vi "Convert Relative Path.vi"(8 "error in (no error)":errorcluster, 10 "File Path in":path, 11 "Report Plugin.lvclass 2":refnum<class "Report Plugin.lvclass">) -> (0 "error out":errorcluster, 2 "Modified Path":path, 3 "Report Plugin.lvclass":refnum<class "Report Plugin.lvclass">)   [LabVIEW 2020]
doc: "If a relative path, convert to the full directory.\n\n<b>Developed by:</b>\nDaniel Coons, TSC"
uses:
  Framework/Report Plugin/Report Plugin.lvclass
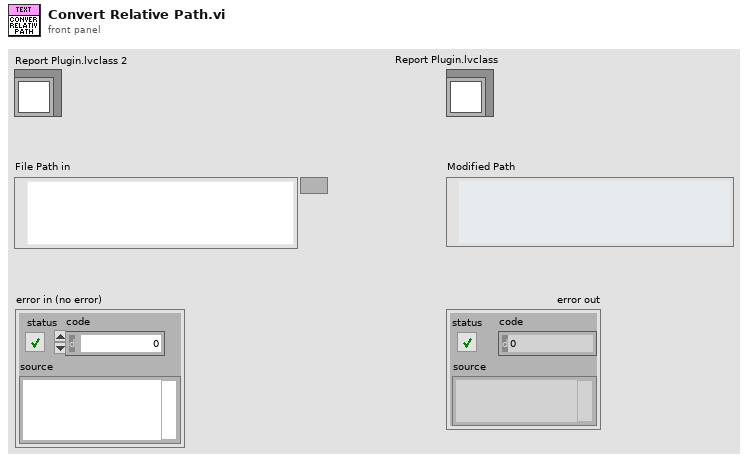
[diagram p1: front panel]
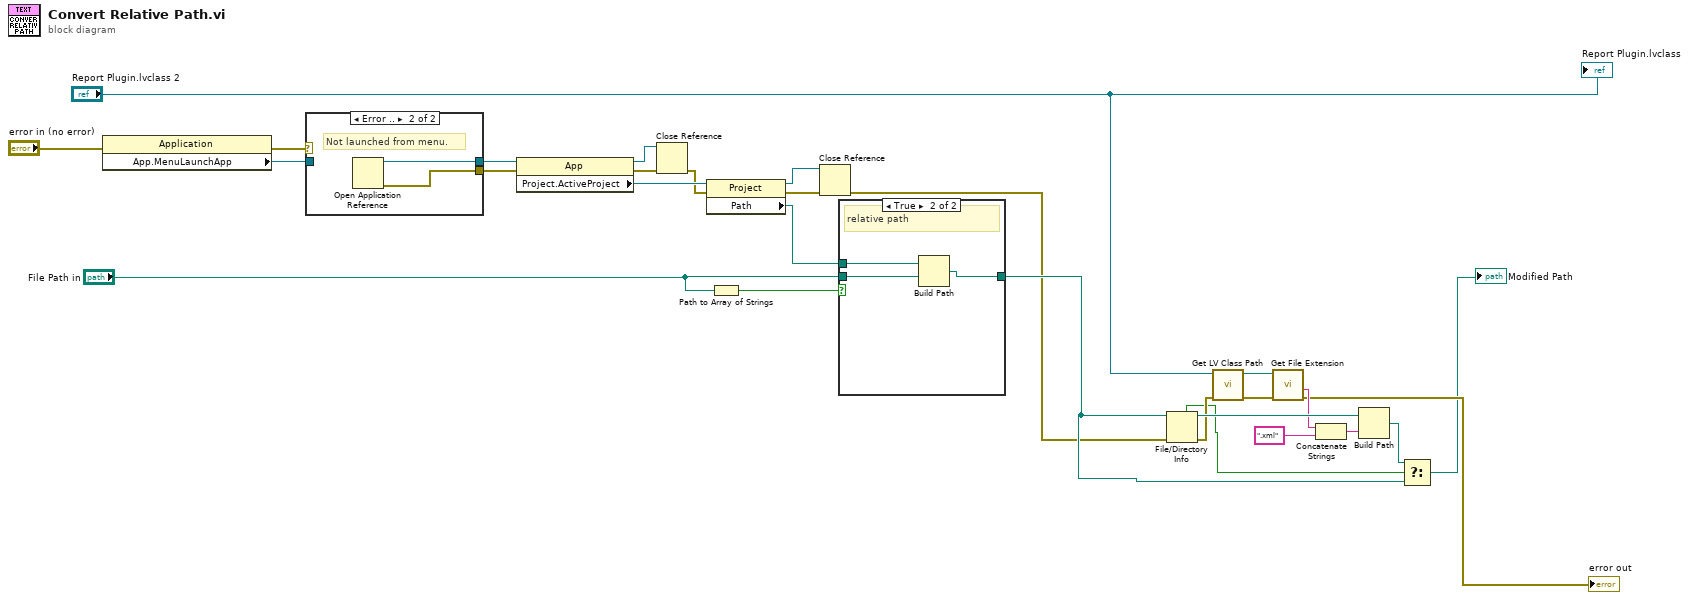
[diagram p0: block diagram]
diagram:
  n1 = property class="Application"(error in="error in (no error)") -> (error out=w16:errorcluster, "App.MenuLaunchApp"=w17:refnum<vi>)  [unwired: 1 in, 1 out]
  n2 = case shown="Error .." w16 {
    selector: w16 -> [w29 _]
    tunnel: [w30 w32] -> w19
    tunnel: w17 -> [w30 _]
    tunnel: [w29 w31] -> w22
    frame No Error {
      # "Launch from menu"
    }
    frame Error {
      # "Not launched from menu."
      n3 = Open Application Reference() -> (0:w31:errorcluster, 3:w32:refnum<vi>)  [unwired: 4 in]
    }
  }
  n4 = property class="App"(reference=w19, error in=w22) -> (reference out=w21:refnum<vi>, error out=w23:errorcluster, "Project.ActiveProject"=w20:refnum<vi>)
  n5 = Close Reference(reference=w21, error in (no error)=w23) -> (error out=w18:errorcluster)
  n6 = property class="Project"(reference=w20, error in=w18) -> (reference out=w24:refnum<vi>, error out=w25:errorcluster, "Path"=w26:path)
  n7 = Path to Array of Strings(0:"File Path in") -> (1:w28:bool)  [unwired: 1 out]
  n8 = Close Reference(reference=w24, error in (no error)=w25) -> (error out=w1:errorcluster)
  n9 = case shown="True" w28 {
    tunnel: "File Path in" -> [w33 w34]
    tunnel: [w33 w35] -> w2
    tunnel: w26 -> [_ w36]
    frame False {
      # "absolute path"
    }
    frame True {
      # "relative path"
      n10 = Build Path(base path=w36, name or relative path=w34) -> (appended path=w35:path)
    }
  }
  n11 = File/Directory Info(path=w2, error in=w1) -> (path out=w15:path, directory=w7:bool, error out=w14:errorcluster)  [unwired: 4 out]
  n12 = call <vilib>:"Get LV Class Path.vi"("error in (no error)"=w14, "object"="Report Plugin.lvclass 2") -> ("error out"=w13:errorcluster, "class path"=w12:path)  [unwired: 8 in]
  n13 = call <vilib>:"Get File Extension.vi"("error in (no error)"=w13, "file"=w12) -> ("error out"=→"error out":errorcluster, "filename without extension"=w11:string)  [unwired: 5 in, 3 out]
  n14 = Concatenate Strings(w11, ".xml" ("string")) -> (w9:string)
  n15 = Build Path(base path=w15, name or relative path=w9) -> (appended path=w8:path)
  n16 = Select(t=w8, s=w7, f=w2) -> (s? t:f=→"Modified Path":path)
  "Report Plugin.lvclass" <- "Report Plugin.lvclass 2"
